vi "scanRegionLogic.vi"(11 "VoltOrScaler?":bool) -> (0 "Error":bool)   [LabVIEW 2014]
uses:
  <vilib>/rvi/Emulation/niFpgaGetClockAttributes.vi
  <vilib>/rvi/Emulation/niFpgaSctlEmulationGetInTimedLoop.vi
  <vilib>/rvi/Emulation/niFpgaEmulationReportErrorSimple.vi
  trackGlobVar.vi
  sequencerGlobVars.vi
  <vilib>/rvi/Emulation/niFpgaCriticalErrorInLSC.vi
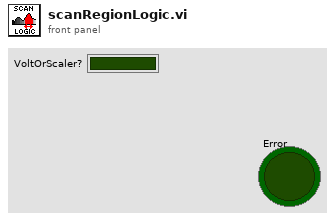
[diagram p1: front panel]
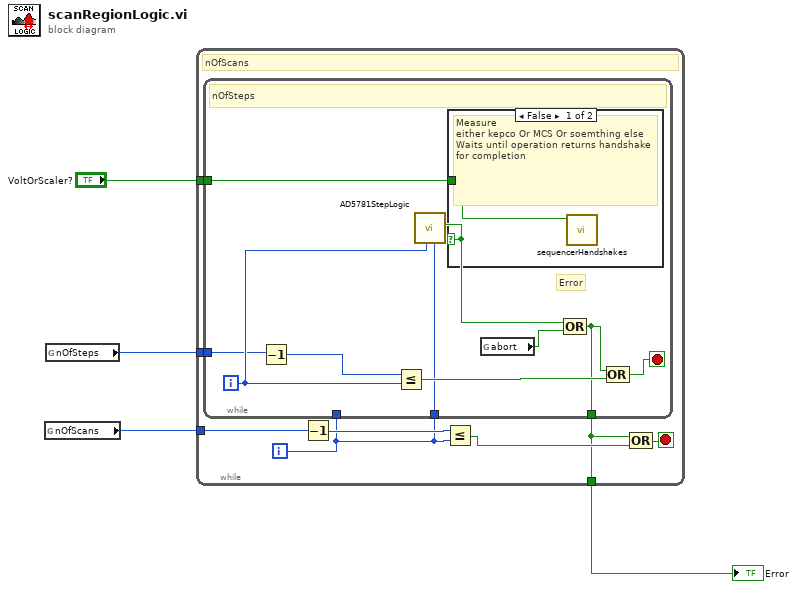
[diagram p0: block diagram]
diagram:
  n1 = global read "trackGlobVar.vi" "nOfScans"() -> (w3:i32)
  n2 = global read "trackGlobVar.vi" "nOfSteps"() -> (w2:i32)
  n3 = while {
    tunnel: [w9] -> w4
    tunnel: w3 -> [w7]
    tunnel: w2 -> [w6]
    tunnel: "VoltOrScaler?" -> [w5]
    i -> [w8]
    stop <- w11 stop-if-true
    # "nOfScans"
    n4 = while {
      tunnel: [w17] -> w9
      tunnel: w8 -> [_]
      tunnel: w8 -> [w15]
      tunnel: w6 -> [w14]
      tunnel: w5 -> [w13]
      i -> [w16]
      stop <- w19 stop-if-true
      # "Error"
      # "nOfSteps"
      n5 = Decrement(x=w14) -> (x-1=w22:i32)
      n6 = Less Or Equal?(x=w22, y=w16) -> (x <= y?=w18:bool)
      n7 = call "AD5781StepLogic.vi"("actTrack"=w15, "actStep"=w16) -> ("timedOut"=w21:bool)  [unwired: 9 in]
      n8 = case shown="False" w21 {
        tunnel: w13 -> [w23 _]
        frame False {
          # "Measure\neither kepco Or MCS Or soemthing else\nWaits until operation returns handshake for completion"
          n9 = call "sequencerHandshakes.vi"("VoltOrScaler?"=w23) -> ()  [unwired: 11 in]
        }
        frame True {
          # "timedOut"
        }
      }
      n10 = global read "sequencerGlobVars.vi" "abort"() -> (w20:bool)
      n11 = Compound Arithmetic op=OR(w21, w20) -> (w17:bool)
      n12 = Compound Arithmetic op=OR(w17, w18) -> (w19:bool)
    }
    n13 = Decrement(x=w7) -> (x-1=w10:i32)
    n14 = Less Or Equal?(x=w10, y=w8) -> (x <= y?=w12:bool)
    n15 = Compound Arithmetic op=OR(w9, w12) -> (w11:bool)
  }
  "Error" <- w4
